vi "Webcam AE.vi"(3 "error in (no error)":errorcluster, 4 "Session In":T3, 5 "Camera states":T1) -> (0 "error out":errorcluster, 1 "Session Out":T3, 2 "Image Out":T2)   [LabVIEW 2018]
uses:
  <vilib>/userdefined/High Color/IMAQdx.ctl
  <vilib>/vision/Image Controls.llb/IMAQ Image.ctl
  Webcam AE.ctl
  <vilib>/vision/driver/IMAQdx.llb/IMAQdx Acquisition Mode.ctl
  <vilib>/vision/driver/IMAQdx.llb/IMAQdx Buffer Number Mode.ctl
  <vilib>/vision/driver/NI_Vision_Acquisition_Software.lvlib
panel:
  out "Image":T2(plugin-control)
  out "Frame Rate":dbl(knob)=9.0 scale=0.0..100.0
  out "Buffer Number":u32=479
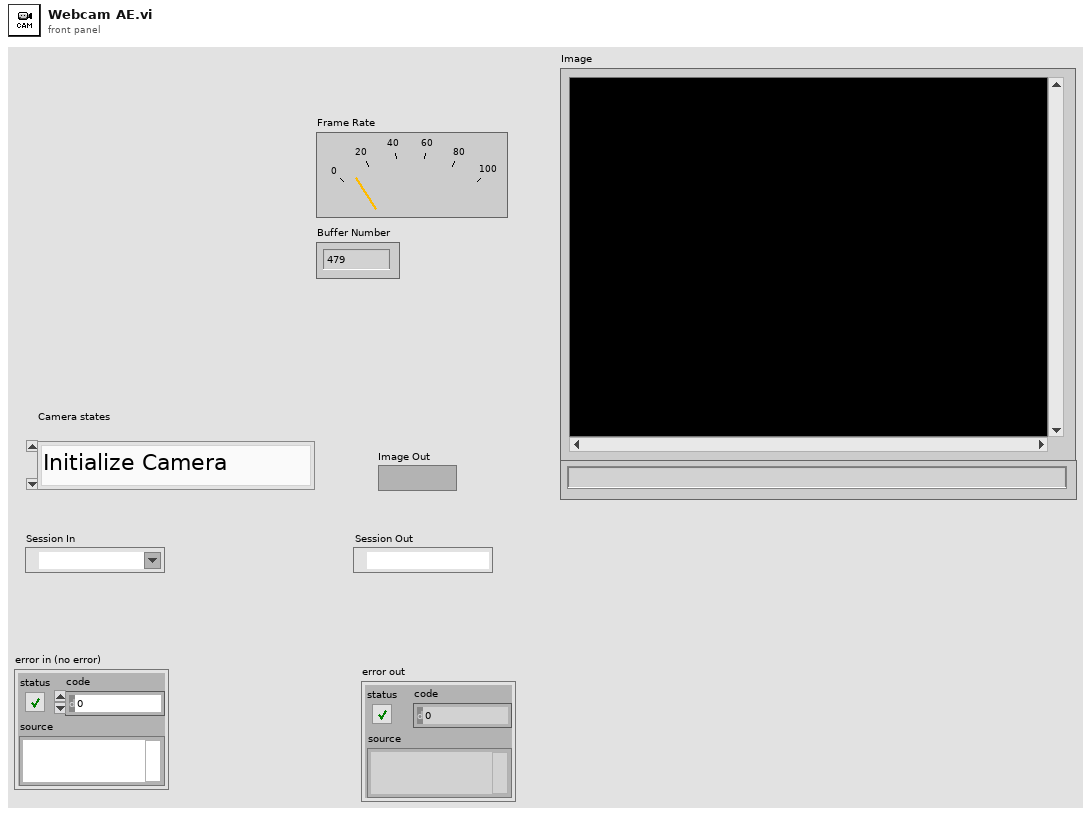
[diagram p1: front panel]
types:
  T1 = typedef "Webcam AE.ctl" = enum16{"Initialize Camera", "Open Camera", "Continuous Acquisition", "Close Camera", "Retrieve Image", "Dispose Camera Image Buffer"}
  T2 = typedef "IMAQ Image.ctl" = refnum<image>
  T3 = typedef "IMAQdx.ctl" = refnum<k21>
  T4 = typedef "NI_Vision_Acquisition_Software.lvlib/IMAQdx Acquisition Mode.ctl" = enum32{"One Shot", "Continuous"}
  T5 = typedef "NI_Vision_Acquisition_Software.lvlib/IMAQdx Buffer Number Mode.ctl" = enum32{"Next", "Last", "Buffer Number", "Every", "Last New"}
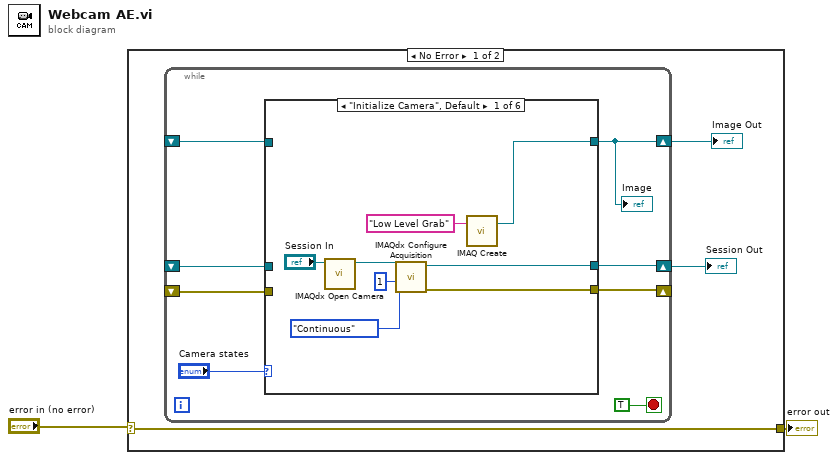
[diagram p0: block diagram]
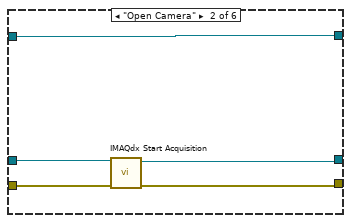
[diagram p2: hidden frame]
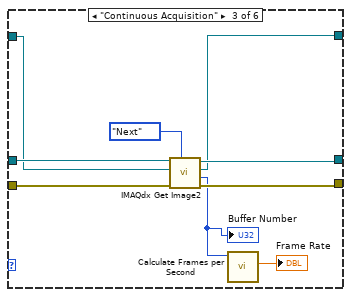
[diagram p3: hidden frame]
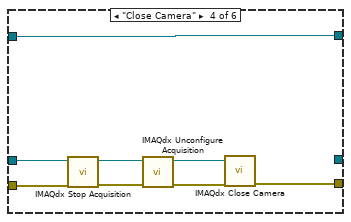
[diagram p4: hidden frame]
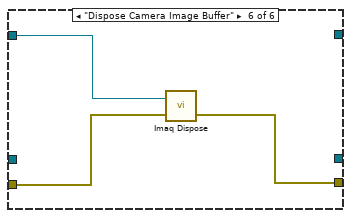
[diagram p6: hidden frame]
diagram:
  n1 = case shown="No Error" "error in (no error)" {
    selector: "error in (no error)" -> [w5 w50]
    tunnel: [w5 w50] -> w1
    frame No Error {
      n2 = while {
        shift-right: [w6] -> w4
        shift-left: _ -> [w8]
        shift-right: [w12] -> w3
        shift-left: _ -> [w10]
        shift-right: [w11] -> _
        shift-left: _ -> [w9]
        stop <- TRUE stop-if-true
        n3 = case shown="\"Initialize Camera\", Default" "Camera states" {
          tunnel: [w17 w23 w31 _ w44 _] -> w12
          tunnel: [w16 w22 w30 w36 w46 w47] -> w11
          tunnel: [w14 w24 w29 w41 w45 _] -> w6
          tunnel: w10 -> [_ w26 w35 w43 w44 _]
          tunnel: w9 -> [_ w25 w34 w42 w46 w48]
          tunnel: w8 -> [_ w24 w33 w41 w45 w49]
          frame "Initialize Camera", Default {
            n4 = call <vilib>:"IMAQdx Open Camera.vi"("Session In"="Session In") -> ("Session Out"=w18:T3)  [unwired: 9 in, 1 out]
            n5 = call <vilib>:"IMAQdx Configure Acquisition.vi"("Number of Buffers"=u32 1, "Continuous?"=IMAQdx_Acquisition_Mode."Continuous", "Session In"=w18) -> ("error out"=w16:errorcluster, "Session Out"=w17:T3)  [unwired: 7 in]
            n6 = call "IMAQ Create"("Image Name"="Low Level Grab") -> ("New Image"=w14:T2)  [unwired: 3 in, 2 out]
          }
          frame "Open Camera" {
            n7 = call <vilib>:"IMAQdx Start Acquisition.vi"("error in"=w25, "Session In"=w26) -> ("error out"=w22:errorcluster, "Session Out"=w23:T3)  [unwired: 8 in]
          }
          frame "Continuous Acquisition" {
            n8 = call <vilib>:"IMAQdx Get Image2.vi"("Buffer Number Mode (Next)"=IMAQdx_Buffer_Number_Mode."Next", "error in"=w34, "Image In"=w33, "Session In"=w35) -> ("error out"=w30:errorcluster, "Buffer Number Out"=w27:u32, "Image Out"=w29:T2, "Session Out"=w31:T3)  [unwired: 4 in]
            "Buffer Number" <- w27
            n9 = call <vilib>:"Calculate Frames per Second.vi"("Buffer Number"=w27) -> ("Processed Frames/s"=→"Frame Rate":dbl)  [unwired: 8 in, 2 out]
          }
          frame "Close Camera" {
            n10 = call <vilib>:"IMAQdx Stop Acquisition.vi"("error in"=w42, "Session In"=w43) -> ("error out"=w39:errorcluster, "Session Out"=w40:T3)  [unwired: 8 in]
            n11 = call <vilib>:"IMAQdx Unconfigure Acquisition.vi"("error in"=w39, "Session In"=w40) -> ("error out"=w37:errorcluster, "Session Out"=w38:T3)  [unwired: 8 in]
            n12 = call <vilib>:"IMAQdx Close Camera.vi"("error in"=w37, "Session In"=w38) -> ("error out"=w36:errorcluster)  [unwired: 9 in]
          }
          frame "Retrieve Image" {
          }
          frame "Dispose Camera Image Buffer" {
            n13 = call "Imaq Dispose"("Image"=w49, "error in (no error)"=w48) -> ("error out"=w47:errorcluster)  [unwired: 4 in]
          }
        }
        "Image" <- w6
      }
      "Image Out" <- w4
      "Session Out" <- w3
    }
    frame Error {
    }
  }
  "error out" <- w1
